vi "Scaling.vi"(8 "error in":errorcluster, 9 "max":dbl, 10 "min":dbl, 11 "value":dbl) -> (0 "error out":errorcluster, 3 "Length out":dbl)   [LabVIEW 2012, in "Spinner.xctl"]
uses:
  Spinner.xctl
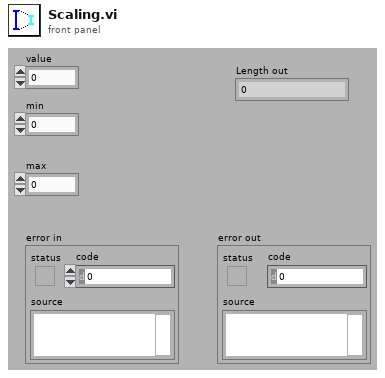
[diagram p1: front panel]
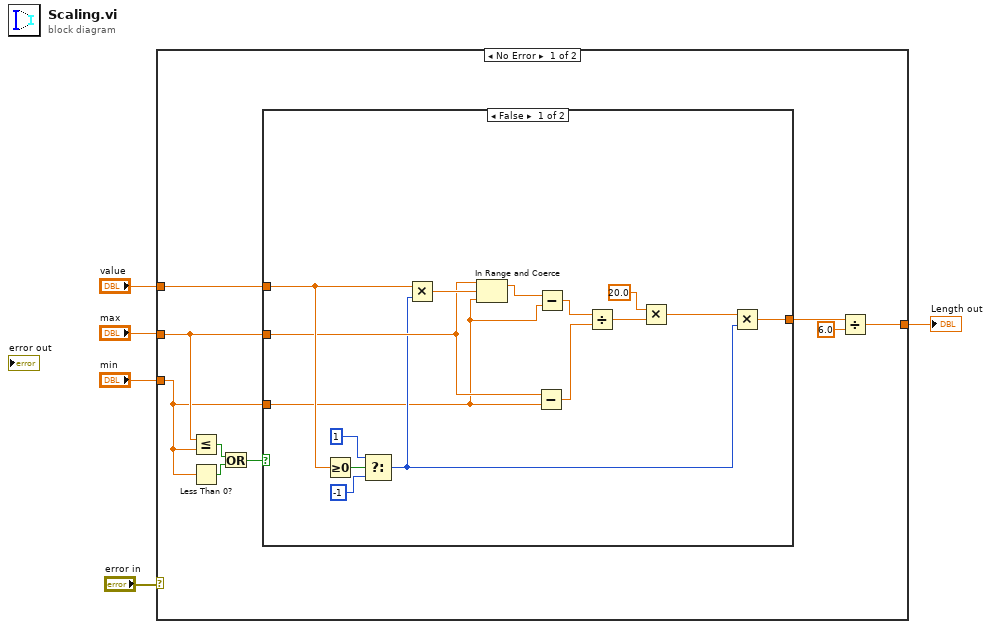
[diagram p0: block diagram]
diagram:
  n1 = case shown="No Error" "error in" {
    tunnel: "max" -> [w13 _]
    tunnel: "min" -> [w12 _]
    tunnel: "value" -> [w9 _]
    tunnel: [w6 _] -> w2
    frame No Error {
      n2 = Less Or Equal?(x=w13, y=w12) -> (x <= y?=w14:bool)
      n3 = Less Than 0?(x=w12) -> (x < 0?=w11:bool)
      n4 = Or(x=w14, y=w11) -> (x .or. y?=w10:bool)
      n5 = case shown="False" w10 {
        tunnel: [w17 _] -> w8
        tunnel: w9 -> [w21 _]
        tunnel: w13 -> [w19 _]
        tunnel: w12 -> [w16 _]
        frame False {
          n6 = Greater Or Equal To 0?(x=w21) -> (x >= 0?=w22:bool)
          n7 = Select(t=1, s=w22, f=-1) -> (s? t:f=w18:i32)
          n8 = Multiply(x=w21, y=w18) -> (x*y=w23:dbl)
          n9 = In Range and Coerce(upper limit=w19, x=w23, lower limit=w16) -> (coerced(x)=w20:dbl)  [unwired: 1 out]
          n10 = Subtract(x=w19, y=w16) -> (x-y=w26:dbl)
          n11 = Subtract(x=w20, y=w16) -> (x-y=w27:dbl)
          n12 = Divide(x=w27, y=w26) -> (x/y=w25:dbl)
          n13 = Multiply(x=20.0 ("y"), y=w25) -> (x*y=w15:dbl)
          n14 = Multiply(x=w15, y=w18) -> (x*y=w17:dbl)
        }
        frame True {
        }
      }
      n15 = Divide(x=w8, y=6.0) -> (x/y=w6:dbl)
    }
    frame Error {
    }
  }
  "Length out" <- w2
